vi "Start Acquisition.vi"(8 "error in (no error)":errorcluster, 11 "Image Acquisition in":refnum<class "HAMAMATSU_DCAMAPI.lvclass">) -> (0 "error out":errorcluster, 3 "Image Acquisition out":refnum<class "HAMAMATSU_DCAMAPI.lvclass">)   [LabVIEW 2020, in "HAMAMATSU_DCAMAPI.lvclass"]
uses:
  HAMAMATSU_DCAMAPI.lvclass
  HAMAMATSU_DCAMAPI.lvclass/HAMAMATSU_DCAMAPI.ctl
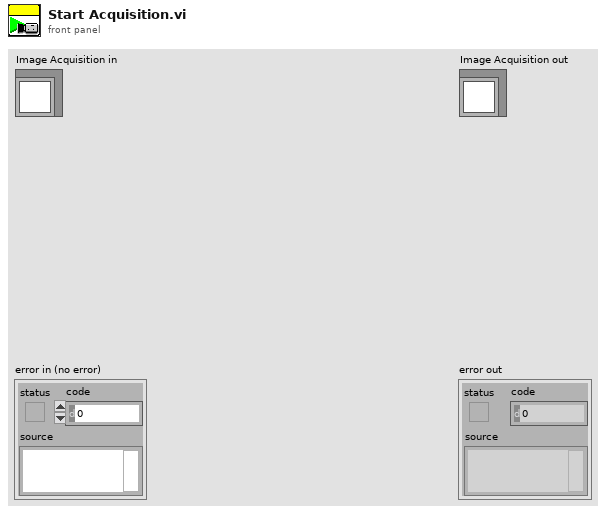
[diagram p1: front panel]
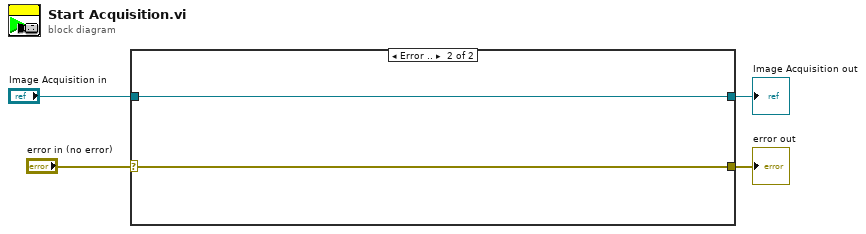
[diagram p0: block diagram]
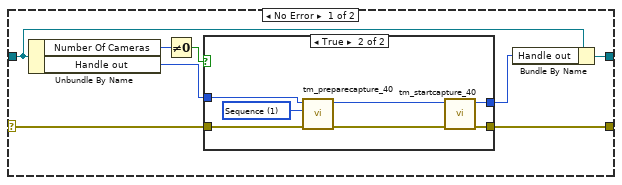
[diagram p2: hidden frame]
diagram:
  n1 = case shown="Error .." "error in (no error)" {
    selector: "error in (no error)" -> [w8 w22]
    tunnel: "Image Acquisition in" -> [w7 w21]
    tunnel: [w9 w22] -> w2
    tunnel: [w5 w21] -> w1
    frame No Error {
      n2 = Unbundle By Name(w7) -> ("Number Of Cameras"=w12:u32, "Handle out"=w10:u32)
      n3 = Not Equal To 0?(x=w12) -> (x != 0?=w11:bool)
      n4 = case shown="True" w11 {
        tunnel: w10 -> [_ w18]
        tunnel: [w13 w16] -> w9
        tunnel: w8 -> [w13 w15]
        tunnel: [_ w14] -> w6
        frame False {
        }
        frame True {
          w17 = 1 items=["Snap", "Sequence"] ("Capture mode")
          n5 = call <userlib>:"tm_preparecapture_40.vi"("error in (no error)"=w15, "Capture mode"=w17, "Handle in"=w18) -> ("error out"=w19:errorcluster, "Handle out"=w20:u32)  [unwired: 5 in, 2 out]
          n6 = call <userlib>:"tm_startcapture_40.vi"("error in (no error)"=w19, "Handle in"=w20) -> ("error out"=w16:errorcluster, "Handle out"=w14:u32)  [unwired: 8 in]
        }
      }
      n7 = Bundle By Name(cluster=w7, "Handle out"=w6) -> (w5:refnum<class "HAMAMATSU_DCAMAPI.lvclass">)
    }
    frame Error {
    }
  }
  "error out" <- w2
  "Image Acquisition out" <- w1
